vi "SinRootSubVi.vi"(0 "x node":i32, 1 "y node":i32, 2 "time":dbl, 3 "u":dbl, 4 "A":dbl, 5 "w":dbl, 6 "x":dbl, 7 "L":dbl) -> (14 "SinRoot":dbl, 18 "SinPart":dbl, 19 "sqrtPart":dbl)   [LabVIEW 2017]
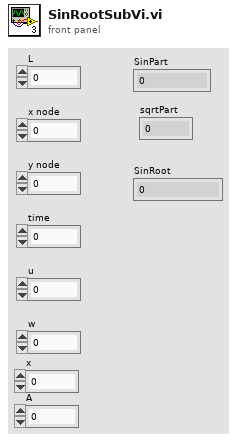
[diagram p1: front panel]
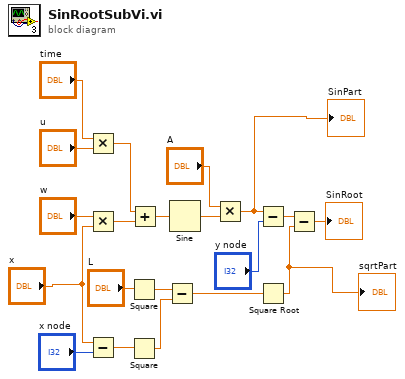
[diagram p0: block diagram]
diagram:
  n1 = Multiply(x="time", y="u") -> (x*y=w14:dbl)
  n2 = Multiply(x="w", y="x") -> (x*y=w13:dbl)
  n3 = Subtract(x="x", y="x node") -> (x-y=w10:dbl)
  n4 = Square(x="L") -> (x^2=w5:dbl)
  n5 = Square(x=w10) -> (x^2=w4:dbl)
  n6 = Add(x=w14, y=w13) -> (x+y=w12:dbl)
  n7 = Subtract(x=w5, y=w4) -> (x-y=w6:dbl)
  n8 = Sine(x=w12) -> (sin(x)=w8:dbl)
  n9 = Multiply(x="A", y=w8) -> (x*y=w3:dbl)
  "SinPart" <- w3
  n10 = Subtract(x=w3, y="y node") -> (x-y=w11:dbl)
  n11 = Square Root(x=w6) -> (sqrt(x)=w2:dbl)
  "sqrtPart" <- w2
  n12 = Subtract(x=w11, y=w2) -> (x-y=→"SinRoot":dbl)
